vi "Fetch Waveform.vi"(8 "error in (no error)":errorcluster, 11 "IScope in":refnum<class "IScope.lvclass">) -> (0 "error out":errorcluster, 3 "IScope out":refnum<class "IScope.lvclass">)   [LabVIEW 2023, in "IScope.lvclass"]
doc: "Since more than one Channel could be configured for Acquisition one has to specify\nwhich specific channel data to fetch"
uses:
  IScope.lvclass
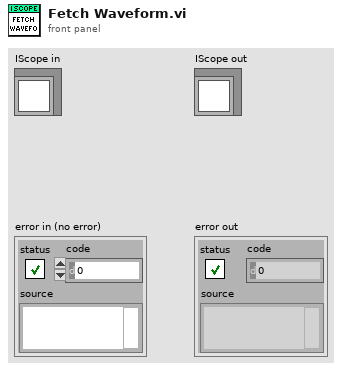
[diagram p1: front panel]
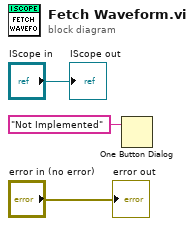
[diagram p0: block diagram]
diagram:
  n1 = One Button Dialog(message="Not Implemented") -> ()  [unwired: 1 in, 1 out]
  "error out" <- "error in (no error)"
  "IScope out" <- "IScope in"
